vi "Set Forward Rotation Direction.vi"(8 "error in (no error)":errorcluster, 10 "forward rotation direction":T1 items=["Clockwise", "Counterclockwise"], 11 "wheel in":refnum<class "NI_Robotics_Wheel.lvclass">) -> (0 "error out":errorcluster, 3 "wheel out":refnum<class "NI_Robotics_Wheel.lvclass">)   [LabVIEW 2017, in "NI_Robotics_Wheel.lvclass"]
uses:
  <vilib>/robotics/Steering/Wheel/NI_Robotics_Wheel.lvclass
  <vilib>/robotics/Steering/Wheel/Rotation Direction.ctl
  <vilib>/robotics/Steering/Wheel/NI_Robotics_Wheel.lvclass/NI_Robotics_Wheel.ctl
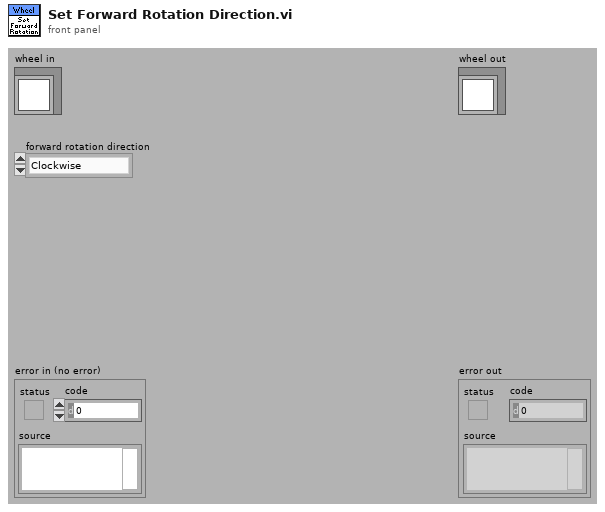
[diagram p1: front panel]
types:
  T1 = typedef "NI_Robotics_Wheel.lvclass/Rotation Direction.ctl" = u16
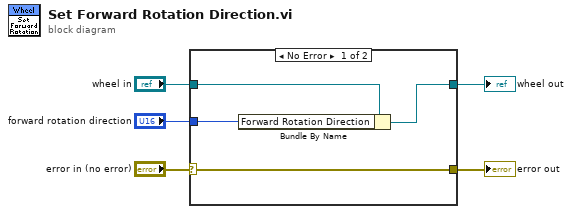
[diagram p0: block diagram]
diagram:
  n1 = case shown="No Error" "error in (no error)" {
    selector: "error in (no error)" -> [w9 w10]
    tunnel: [w9 w10] -> w4
    tunnel: [w7 w11] -> w2
    tunnel: "wheel in" -> [w8 w11]
    tunnel: "forward rotation direction" -> [w6 _]
    frame No Error {
      n2 = Bundle By Name(cluster=w8, "Forward Rotation Direction"=w6) -> (w7:refnum<class "NI_Robotics_Wheel.lvclass">)
    }
    frame Error {
    }
  }
  "error out" <- w4
  "wheel out" <- w2
